vi "XML Script - Build Array.vi"(0 "x":i32=-1, 1 "y":i32=-1, 2 "out":i32=-1, 4 "concat inputs?":bool, 6 "name":string, 8 "size":i32=1, 9 "prefix (name)":string, 10 "in":i32=-1) -> (5 "name (wire source)":string, 7 "XML Script Command - Build Array":string)   [LabVIEW 2020]
uses:
  <vilib>/_script/XML Scripting/XML Script Attribute.ctl
  <vilib>/_script/XML Scripting/XML Script Tag.ctl
panel:
  # "position"
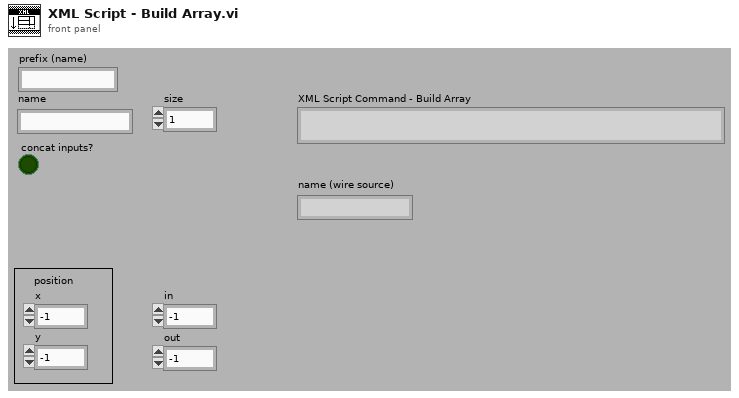
[diagram p1: front panel]
types:
  T1 = typedef "XML Script Attribute.ctl" = enum16{"name", "style", "path", "position", "in", "out", "width", "height", "index", "value", "default", "location", "offset", "typeindex", "size", "source", "destination", "indicator", "type", "controlname", "label", "conpaneidx", "mode", "description", "hasCondTerm", "linkIdentity", "caseselectortype", "concatInputs", "inName", "instantiationpath", "loopCondition", "IndexMode", "formulaInputs", "formulaOutputs", "msnFuncName", "msnIsDynamic", "msnIsODEUserFunction", "ignoreSearchDialog"}
  T2 = typedef "XML Script Tag.ctl" = enum16{"Script", "Function", "SubVI", "GrowableFunction", "Structure", "MultiframeStructure", "Frame", "Tunnel", "ShiftRegister", "Constant", "Control", "Terminal", "Wire", "StaticVIReference", "ControlTerminal", "CompoundArithmetic", "FlatSequence", "FlatSequenceFrame", "MathScriptCallByRef", "BuildArray", "GenericSubVI", "MathScriptNode"}
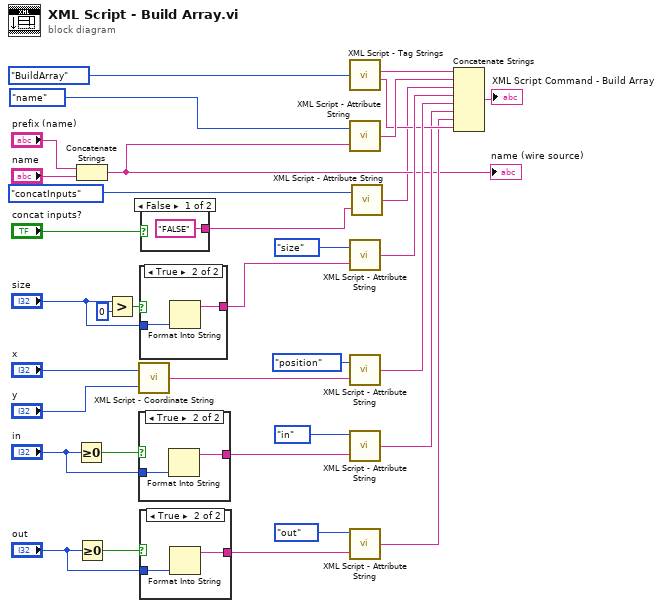
[diagram p0: block diagram]
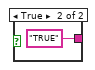
[diagram p2: hidden frame]
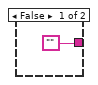
[diagram p3: hidden frame]
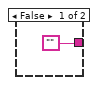
[diagram p4: hidden frame]
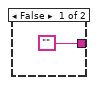
[diagram p5: hidden frame]
diagram:
  n1 = Greater Or Equal To 0?(x="in") -> (x >= 0?=w14:bool)
  n2 = Concatenate Strings("prefix (name)", "name") -> (w5:string)
  "name (wire source)" <- w5
  n3 = Greater Or Equal To 0?(x="out") -> (x >= 0?=w18:bool)
  n4 = Greater?(x="size", y=0) -> (0:w30:bool)
  n5 = call <vilib>:"XML Script - Coordinate String.vi"("y"="y", "x"="x") -> ("(x,y)"=w28:string)
  n6 = case shown="True" w14 {
    tunnel: "in" -> [_ w37]
    tunnel: ["" w36] -> w16
    frame False {
    }
    frame True {
      n7 = Format Into String(w37) -> (resulting string=w36:string)  [unwired: 3 in, 1 out]
    }
  }
  n8 = case shown="True" w30 {
    tunnel: "size" -> [_ w40]
    tunnel: ["" w39] -> w22
    frame False {
    }
    frame True {
      n9 = Format Into String(w40) -> (resulting string=w39:string)  [unwired: 3 in, 1 out]
    }
  }
  n10 = case shown="True" w18 {
    tunnel: "out" -> [_ w43]
    tunnel: ["" w42] -> w20
    frame False {
    }
    frame True {
      n11 = Format Into String(w43) -> (resulting string=w42:string)  [unwired: 3 in, 1 out]
    }
  }
  n12 = case shown="False" "concat inputs?" {
    tunnel: ["FALSE" "TRUE"] -> w3
    frame False {
    }
    frame True {
    }
  }
  n13 = call <vilib>:"XML Script - Tag Strings.vi"("XML Script Tag"=XML_Script_Tag."BuildArray") -> ("XML String - Begin Tag"=w25:string, "XML String - End Tag"=w10:string)  [unwired: 2 out]
  n14 = call <vilib>:"XML Script - Attribute String.vi"("Attribute String"=w5, "XML Script Attribute"=XML_Script_Attribute."name") -> ("XML Script - Attribute String"=w23:string)
  n15 = call <vilib>:"XML Script - Attribute String.vi"("Attribute String"=w22, "XML Script Attribute"=XML_Script_Attribute."size") -> ("XML Script - Attribute String"=w12:string)
  n16 = call <vilib>:"XML Script - Attribute String.vi"("Attribute String"=w28, "XML Script Attribute"=XML_Script_Attribute."position") -> ("XML Script - Attribute String"=w11:string)
  n17 = call <vilib>:"XML Script - Attribute String.vi"("Attribute String"=w16, "XML Script Attribute"=XML_Script_Attribute."in") -> ("XML Script - Attribute String"=w9:string)
  n18 = call <vilib>:"XML Script - Attribute String.vi"("Attribute String"=w20, "XML Script Attribute"=XML_Script_Attribute."out") -> ("XML Script - Attribute String"=w8:string)
  n19 = call <vilib>:"XML Script - Attribute String.vi"("Attribute String"=w3, "XML Script Attribute"=XML_Script_Attribute."concatInputs") -> ("XML Script - Attribute String"=w2:string)
  n20 = Concatenate Strings(w25, w23, w2, w12, w11, w9, w8, w10) -> (→"XML Script Command - Build Array":string)
